vi "Precess.vi"() -> ()   [LabVIEW 2010]
panel:
  in  "EQUINOX 2":dbl format="%<%H:%M:%S>t"
  in  "EQUINOX1":dbl format="%<%H:%M:%S>t"
  in  "DEC":dbl format="%<%H:%M:%S>t"
  in  "RA":dbl format="%<%H:%M:%S>t"
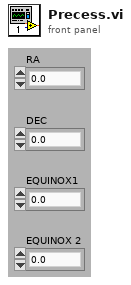
[diagram p1: front panel]
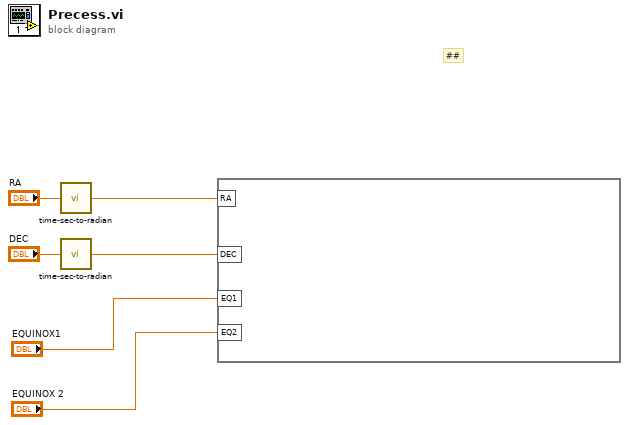
[diagram p0: block diagram]
diagram:
  # "##"
  n1 = call "time-sec-to-radian.vi"("Numeric"="RA") -> ("radians"=w4:dbl)
  n2 = call "time-sec-to-radian.vi"("Numeric"="DEC") -> ("radians"=w3:dbl)
  n3 = formula code=""("RA"=w4, "DEC"=w3, "EQ1"="EQUINOX1", "EQ2"="EQUINOX 2") -> ()
